vi "ALL PROBLEM.vi"() -> ()   [LabVIEW 2017]
panel:
  in  "stop":bool
  out "DANGER":bool
  out "AC":bool
  out "FAN":bool
  in  "Thermometer":dbl(slide) scale=0.0..150.0
  # "AUTOMATED SAFETY MONITERING"
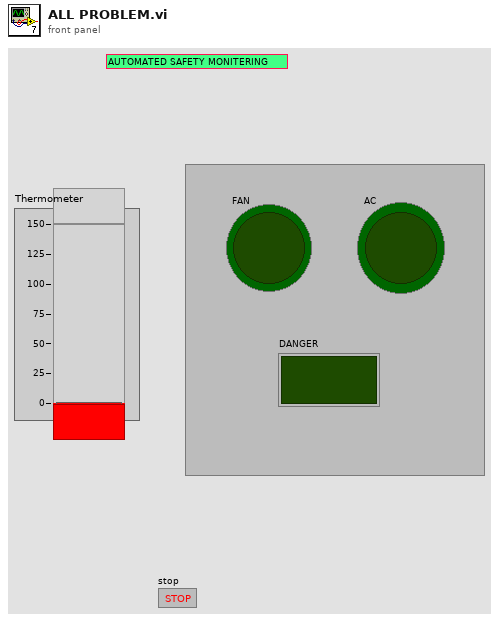
[diagram p1: front panel]
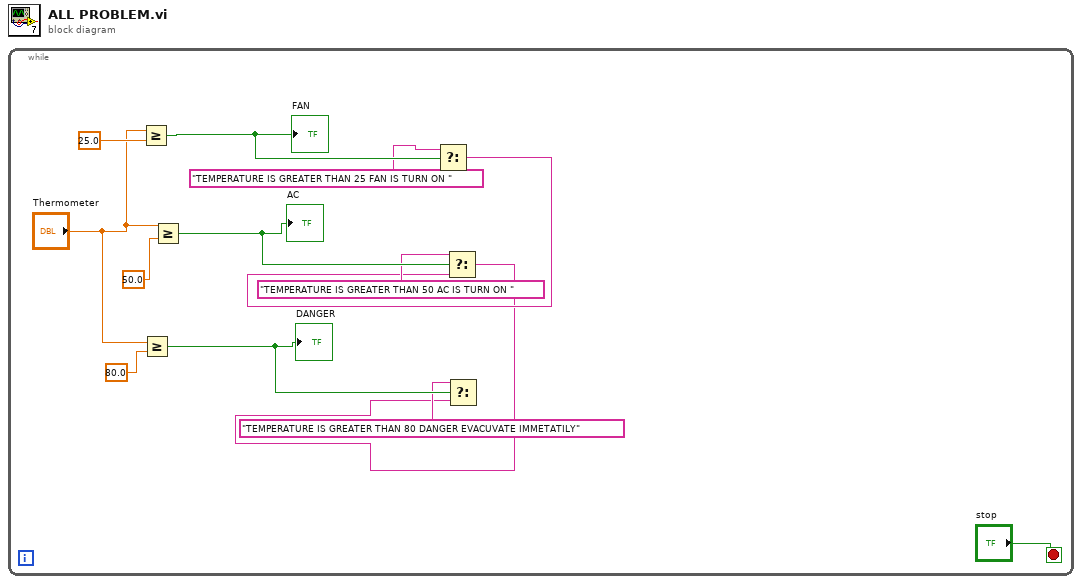
[diagram p0: block diagram]
diagram:
  n1 = while {
    stop <- "stop" stop-if-true
    n2 = Greater Or Equal?(x="Thermometer", y=25.0) -> (x >= y?=w8:bool)
    "FAN" <- w8
    n3 = Greater Or Equal?(x="Thermometer", y=80.0) -> (x >= y?=w6:bool)
    "DANGER" <- w6
    n4 = Greater Or Equal?(x="Thermometer", y=50.0) -> (x >= y?=w7:bool)
    "AC" <- w7
    n5 = Select(t="TEMPERATURE IS GREATER THAN 25 FAN IS TURN ON ", s=w8) -> (s? t:f=w2:string)  [unwired: 1 in]
    n6 = Select(t="TEMPERATURE IS GREATER THAN 50 AC IS TURN ON ", s=w7, f=w2) -> (s? t:f=w1:string)
    n7 = Select(t="TEMPERATURE IS GREATER THAN 80 DANGER EVACUVATE IMMETATILY", s=w6, f=w1) -> ()  [unwired: 1 out]
  }
